vi "parse_dataString.vi"(4 "Timestamp":ext, 6 "Timebase Frequency":ext, 7 "Includes Timestamp?":bool=TRUE, 8 "error in (no error)":errorcluster, 9 "ChannelInfo":T2, 10 "Data Type":u32, 11 "Data String":string) -> (0 "error out":errorcluster, 3 "Data":T1)   [LabVIEW 2020, in "OXYGEN_Datastream.lvlib"]
uses:
  OXYGEN_Datastream.lvlib
  TypeDefs/ChannelInfo.ctl
  TypeDefs/ChannelInfo_Scaling.ctl
  TypeDefs/DataPoint_Variant.ctl
  TypeDefs/CAN_Data.ctl
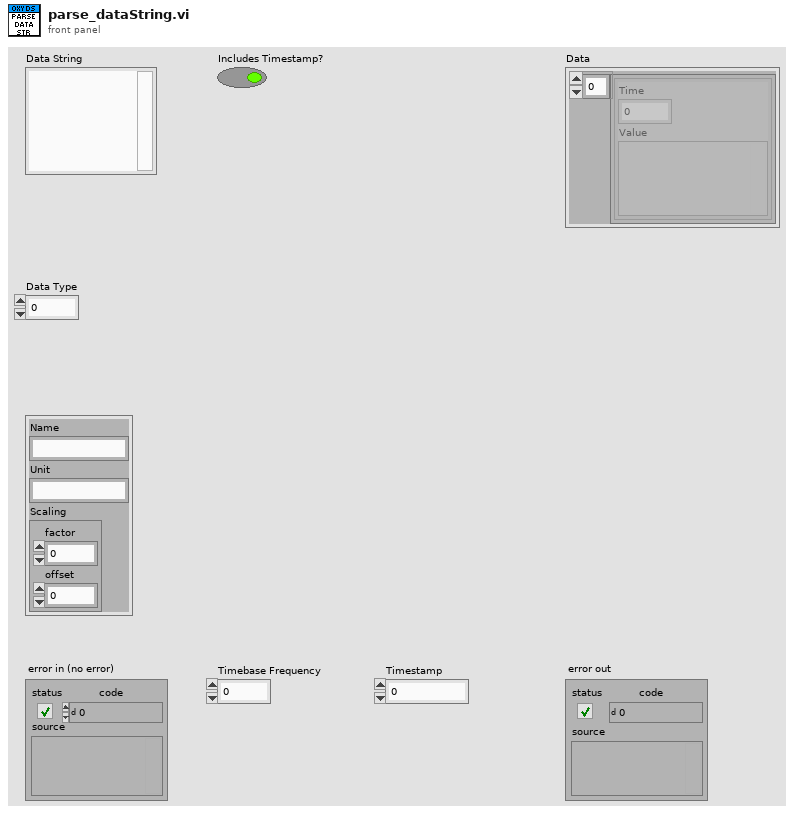
[diagram p1: front panel]
types:
  T1 = typedef "OXYGEN_Datastream.lvlib/DataPoint_Variant.ctl" = cluster{"DataPoints":cluster{"Time":dbl, "Value":variant}[]}
  T2 = typedef "OXYGEN_Datastream.lvlib/ChannelInfo.ctl" = cluster{"Name":string, "Unit":string, "Scaling":T3}
  T3 = typedef "OXYGEN_Datastream.lvlib/ChannelInfo_Scaling.ctl" = cluster{"factor":dbl, "offset":dbl}
  T4 = enum16{"big-endian, network order", "native, host order", "little-endian"}
  T5 = typedef "OXYGEN_Datastream.lvlib/CAN_Data.ctl" = cluster{"ID":string, "Message":string}
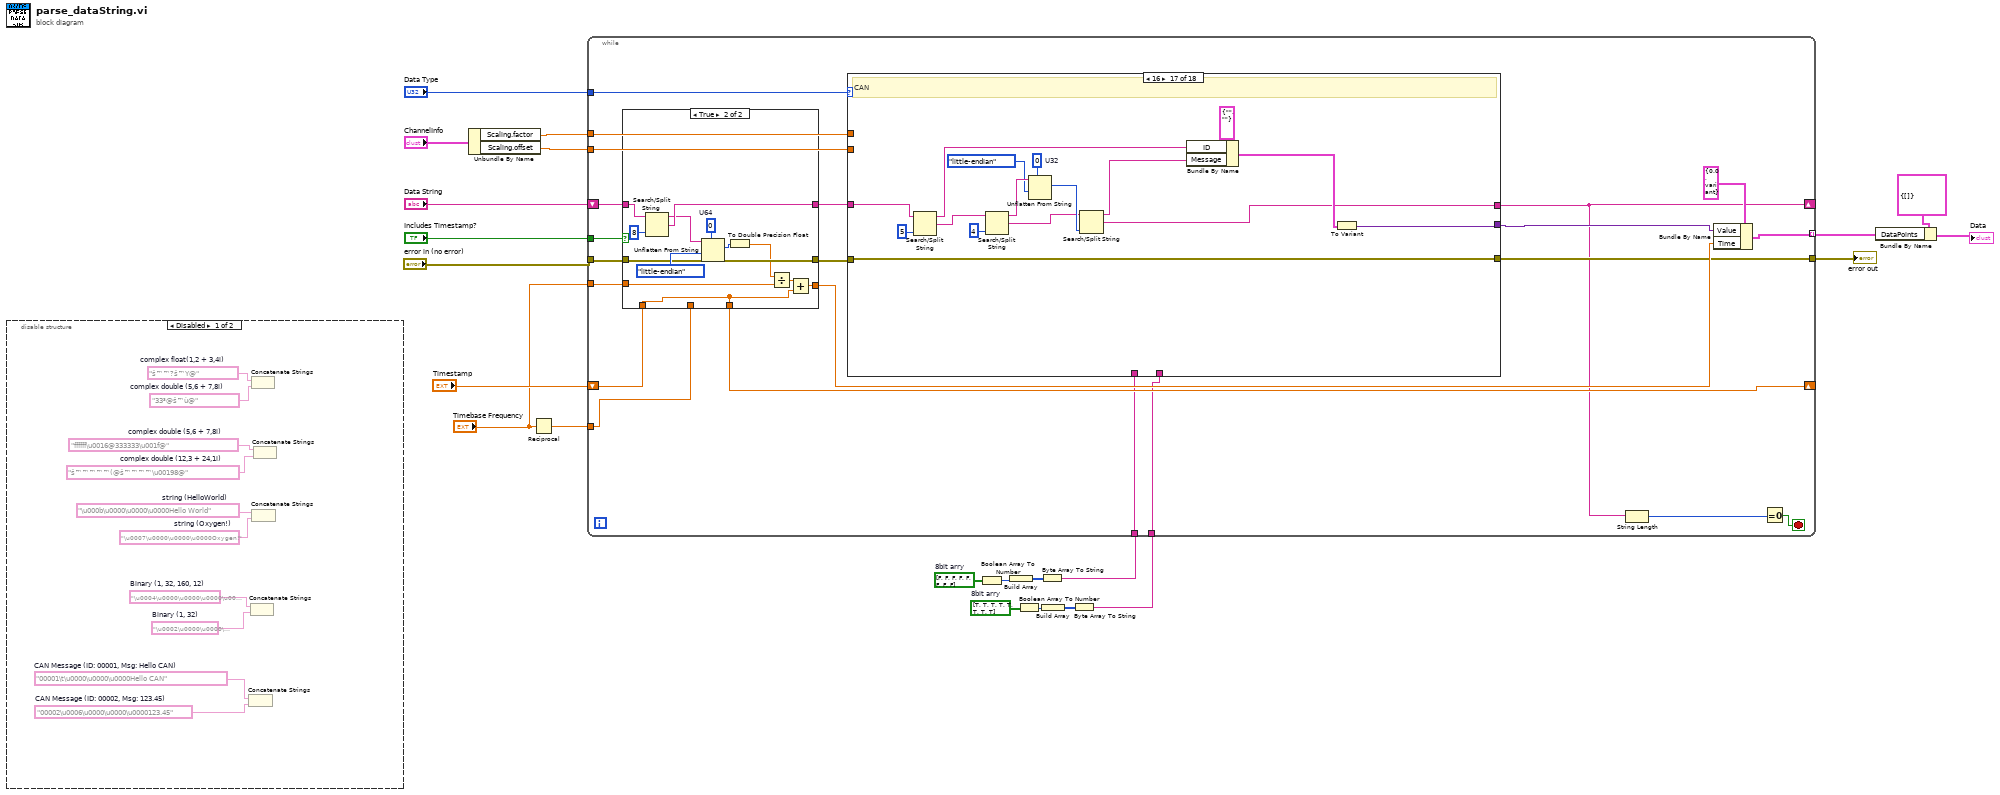
[diagram p0: block diagram]
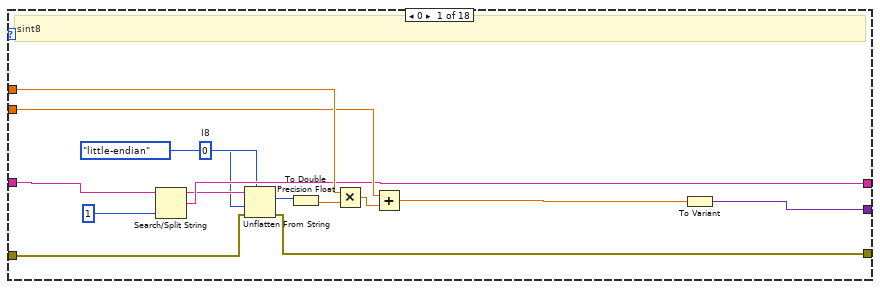
[diagram p3: hidden frame]
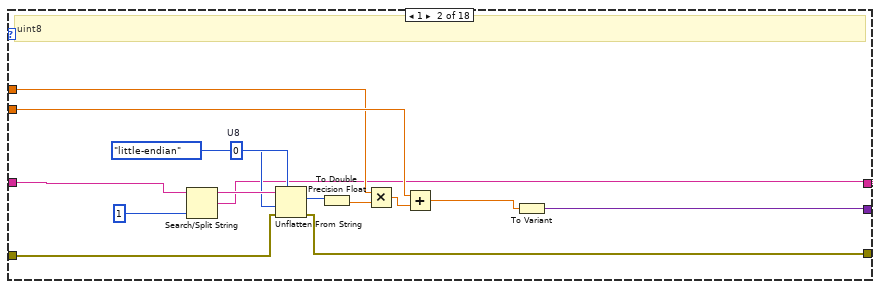
[diagram p4: hidden frame]
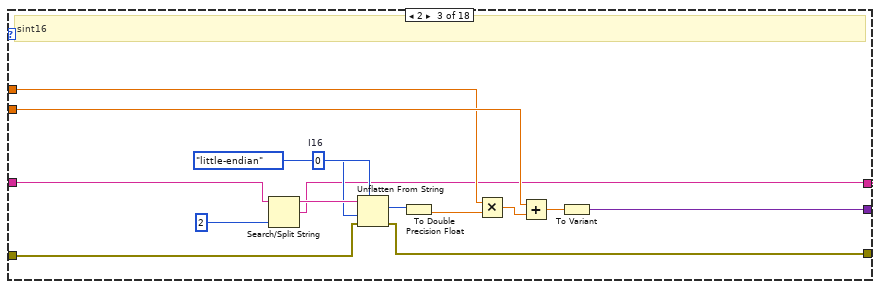
[diagram p5: hidden frame]
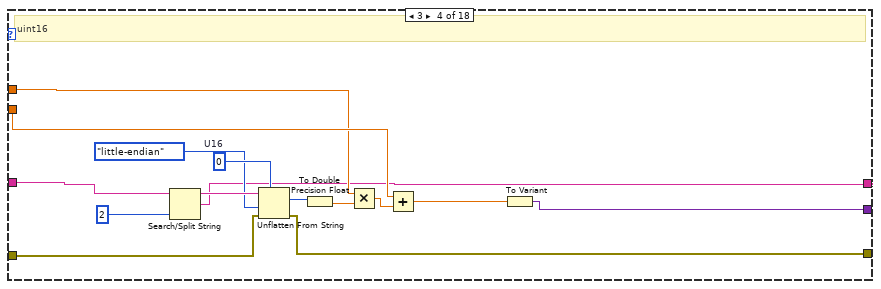
[diagram p6: hidden frame]
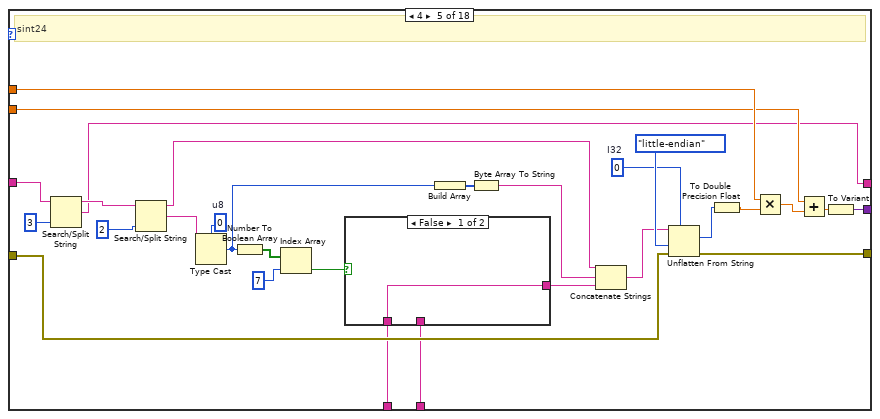
[diagram p7: hidden frame]
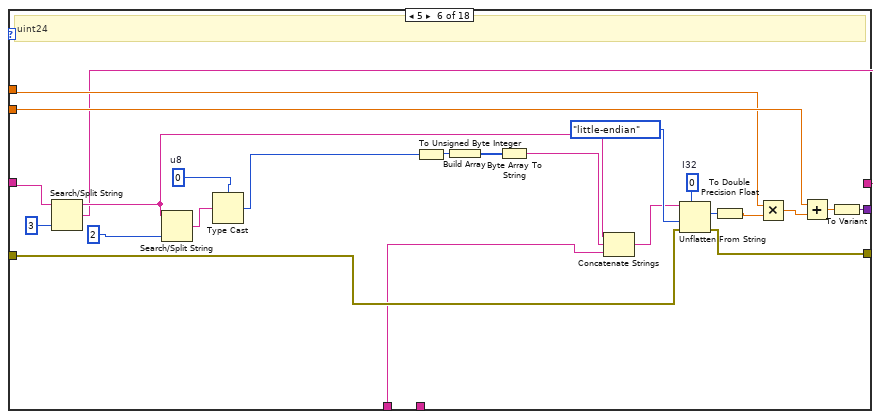
[diagram p9: hidden frame]
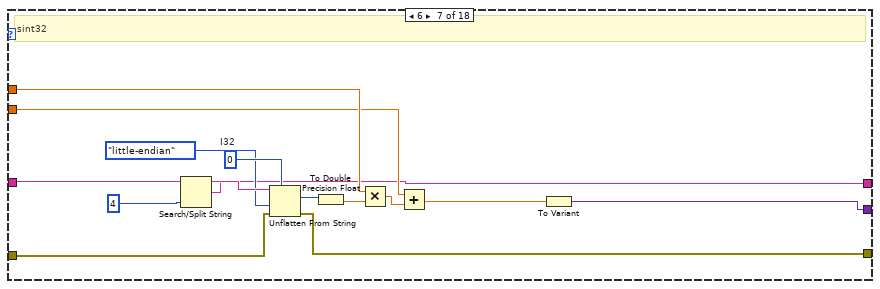
[diagram p10: hidden frame]
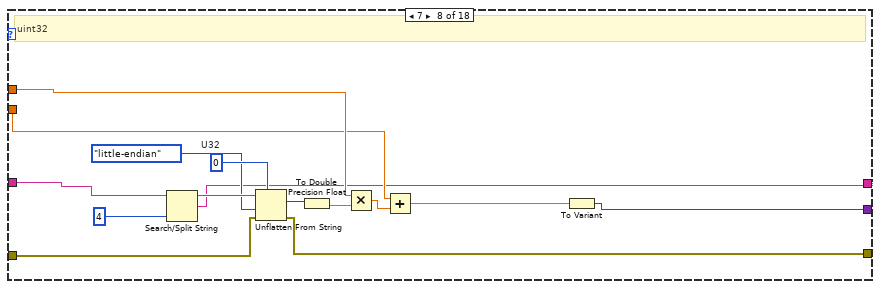
[diagram p11: hidden frame]
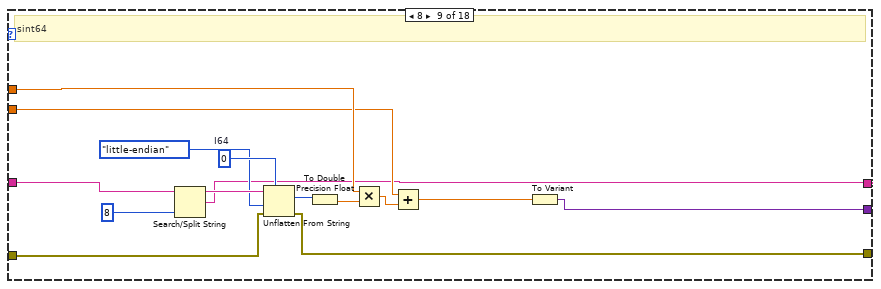
[diagram p12: hidden frame]
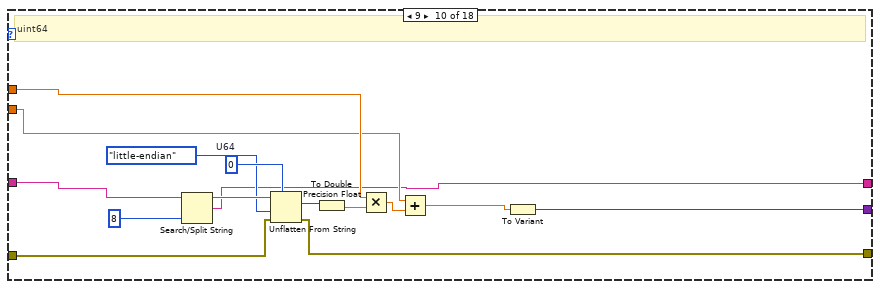
[diagram p13: hidden frame]
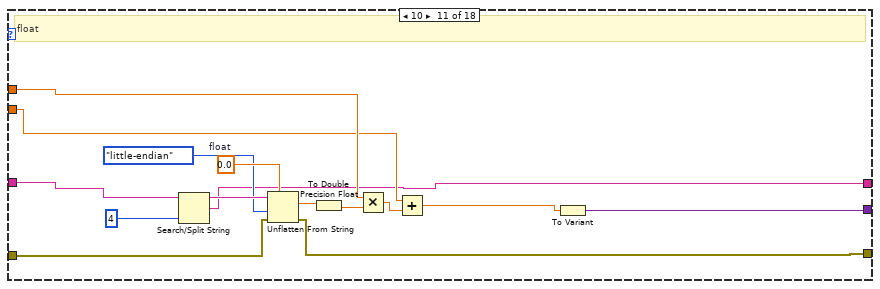
[diagram p14: hidden frame]
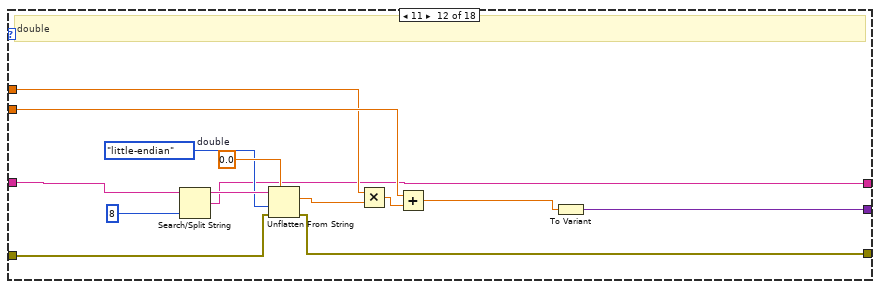
[diagram p15: hidden frame]
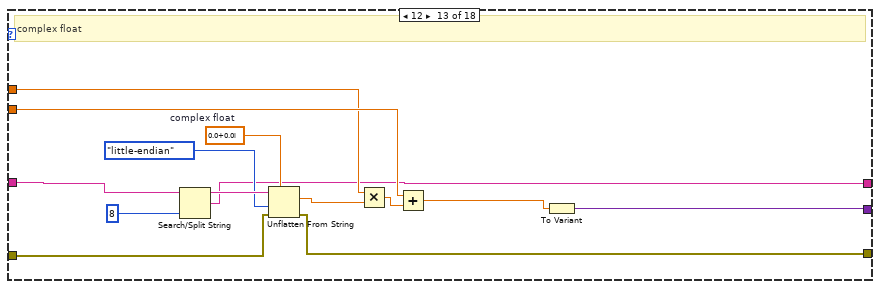
[diagram p16: hidden frame]
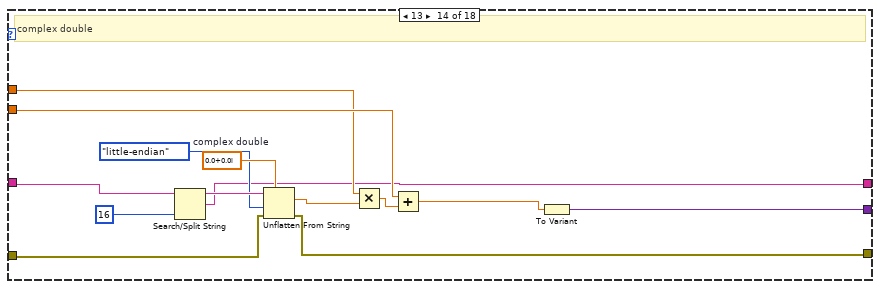
[diagram p17: hidden frame]
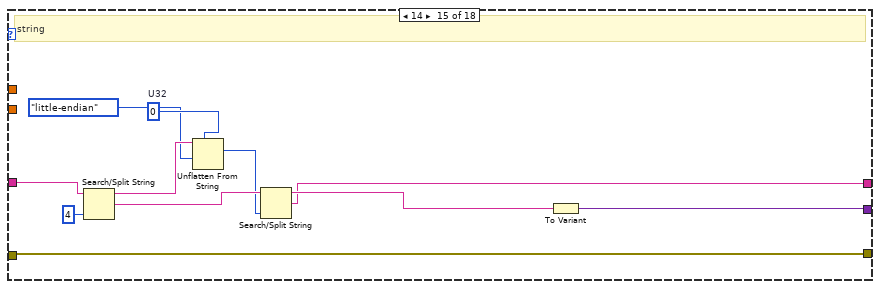
[diagram p18: hidden frame]
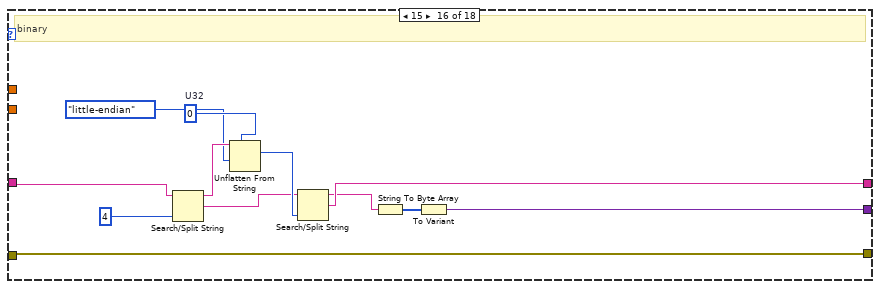
[diagram p19: hidden frame]
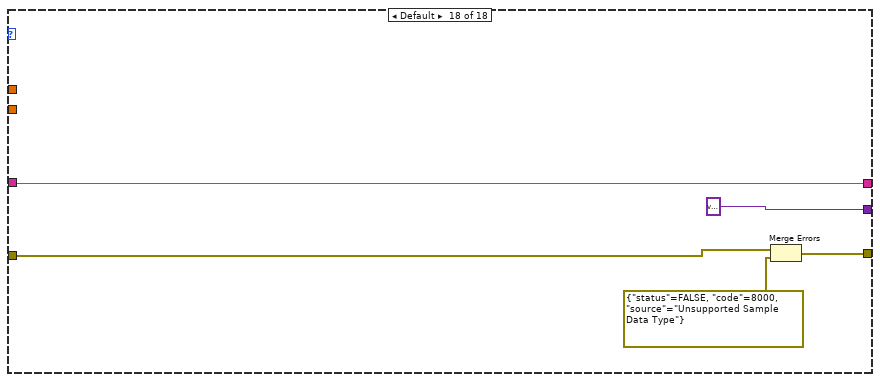
[diagram p20: hidden frame]
diagram:
  w8 = bool[] [TRUE, TRUE, TRUE, TRUE, TRUE, TRUE, TRUE, TRUE]  # 8bit arry
  w9 = bool[] [FALSE, FALSE, FALSE, FALSE, FALSE, FALSE, FALSE, FALSE]  # 8bit arry
  n1 = disable-structure shown="Disabled" {
    frame Disabled {
      w23 = "00002\u0006\u0000\u0000\u0000123.45"  # CAN Message (ID: 00002, Msg: 123.45)
      w24 = "00001\t\u0000\u0000\u0000Hello CAN"  # CAN Message (ID: 00001, Msg: Hello CAN)
      w25 = "\u0002\u0000\u0000\u0000\u0001 "  # Binary (1, 32)
      w26 = "\u0004\u0000\u0000\u0000\u0001  \f"  # Binary (1, 32, 160, 12)
      w27 = "š™™™™™(@š™™™™\u00198@"  # complex double (12,3 + 24,1i)
      w29 = "33³@š™ù@"  # complex double (5,6 + 7,8i)
      w31 = "\u0007\u0000\u0000\u0000Oxygen!"  # string (Oxygen!)
      w32 = "\u000b\u0000\u0000\u0000Hello World"  # string (HelloWorld)
      w28 = "ffffff\u0016@333333\u001f@"  # complex double (5,6 + 7,8i)
      w30 = "š™™?š™Y@"  # complex float(1,2 + 3,4i)
      n2 = Concatenate Strings(w24, w23) -> ()  [unwired: 1 out]
      n3 = Concatenate Strings(w26, w25) -> ()  [unwired: 1 out]
      n4 = Concatenate Strings(w30, w29) -> ()  [unwired: 1 out]
      n5 = Concatenate Strings(w32, w31) -> ()  [unwired: 1 out]
      n6 = Concatenate Strings(w28, w27) -> ()  [unwired: 1 out]
    }
    frame Enabled {
    }
  }
  n7 = Unbundle By Name("ChannelInfo") -> ("Scaling.factor"=w19:dbl, "Scaling.offset"=w18:dbl)
  n8 = Reciprocal(x="Timebase Frequency") -> (1/x=w10:ext)
  n9 = Boolean Array To Number(Boolean array=w9) -> (number=w7:u32)
  n10 = Build Array(w7) -> (w6:u32[])
  n11 = Boolean Array To Number(Boolean array=w8) -> (number=w5:u32)
  n12 = Byte Array To String(unsigned byte array=w6) -> (string=w3:string)
  n13 = Build Array(w5) -> (w4:u32[])
  n14 = Byte Array To String(unsigned byte array=w4) -> (string=w2:string)
  n15 = while {
    tunnel: "Data Type" -> [w39]
    tunnel: w19 -> [w40]
    tunnel: w18 -> [w41]
    shift-right: [w36] -> _
    shift-left: "Data String" -> [w52]
    tunnel: "Includes Timestamp?" -> [w48]
    tunnel: "error in (no error)" -> [w51]
    tunnel: [w38] -> w16
    tunnel: [w49] -> w12 mode=indexing
    shift-right: [w44] -> _
    shift-left: "Timestamp" -> [w47]
    tunnel: w10 -> [w46]
    tunnel: w3 -> [w35]
    tunnel: w2 -> [w34]
    tunnel: "Timebase Frequency" -> [w33]
    stop <- w53 stop-if-true
    n16 = case shown="True" w48 {
      tunnel: w52 -> [w335 w348]
      tunnel: [w335 w347] -> w42
      tunnel: [w332 w338] -> w45
      tunnel: [w334 w342] -> w43
      tunnel: w51 -> [w334 w341]
      tunnel: w47 -> [w332 w337]
      tunnel: w46 -> [w333 _]
      tunnel: [w331 w337] -> w44
      tunnel: w33 -> [_ w336]
      frame False {
        n17 = Add(x=w332, y=w333) -> (x+y=w331:ext)
      }
      frame True {
        w345 = u64 0  # U64
        n18 = Search/Split String(string=w348, offset (0)=8) -> (substring before match=w346:string, match + rest of string=w347:string)  [unwired: 1 in, 1 out]
        n19 = Unflatten From String(type=w345, binary string=w346, byte order (0:big-endian, network order)=T4."little-endian", error in (no error)=w341) -> (value=w343:u64, error out=w342:errorcluster)  [unwired: 1 in, 1 out]
        n20 = To Double Precision Float(number=w343) -> (double precision float=w339:dbl)
        n21 = Divide(x=w339, y=w336) -> (x/y=w340:ext)
        n22 = Add(x=w340, y=w337) -> (x+y=w338:ext)
      }
    }
    n23 = case shown="16" w39 {
      tunnel: w42 -> [w69 w84 w99 w114 w143 w169 w182 w197 w212 w227 w242 w258 w272 w278 w294 w302 w317 w330]
      tunnel: [w55 w70 w85 w100 w121 w151 w171 w185 w200 w215 w230 w245 w259 w274 w297 w298 w313 variant] -> w37
      tunnel: w40 -> [w68 w82 w97 w112 w142 w167 w184 w199 w214 w229 w244 w256 w270 w276 _ _ _ _]
      tunnel: w41 -> [w67 w83 w98 w113 w141 w168 w183 w198 w213 w228 w243 w257 w271 w277 _ _ _ _]
      tunnel: [w66 w74 w89 w104 w125 w155 w174 w189 w204 w219 w234 w249 w263 w275 w287 w301 w311 w330] -> w36
      tunnel: w43 -> [w58 w73 w88 w103 w124 w154 w173 w187 w202 w217 w232 w247 w261 w279 w296 w309 w325 w328]
      tunnel: [w57 w72 w87 w102 w123 w153 w172 w188 w203 w218 w233 w248 w262 w273 w296 w309 w325 w329] -> w38
      tunnel: w35 -> [_ _ _ _ w120 w150 _ _ _ _ _ _ _ _ _ _ _ _]
      tunnel: w34 -> [_ _ _ _ w119 _ _ _ _ _ _ _ _ _ _ _ _ _]
      frame 0 {
        w63 = i8 0  # I8
        # "sint8"
        n24 = Search/Split String(string=w69, offset (0)=1) -> (substring before match=w64:string, match + rest of string=w66:string)  [unwired: 1 in, 1 out]
        n25 = Unflatten From String(type=w63, binary string=w64, byte order (0:big-endian, network order)=T4."little-endian", error in (no error)=w58) -> (value=w61:i8, error out=w57:errorcluster)  [unwired: 1 in, 1 out]
        n26 = To Double Precision Float(number=w61) -> (double precision float=w60:dbl)
        n27 = Multiply(x=w68, y=w60) -> (x*y=w59:dbl)
        n28 = Add(x=w67, y=w59) -> (x+y=w56:dbl)
        n29 = To Variant(anything=w56) -> (Variant=w55:variant)
      }
      frame 1 {
        w79 = u8 0  # U8
        # "uint8"
        n30 = Search/Split String(string=w84, offset (0)=1) -> (substring before match=w80:string, match + rest of string=w74:string)  [unwired: 1 in, 1 out]
        n31 = Unflatten From String(type=w79, binary string=w80, byte order (0:big-endian, network order)=T4."little-endian", error in (no error)=w73) -> (value=w77:u8, error out=w72:errorcluster)  [unwired: 1 in, 1 out]
        n32 = To Double Precision Float(number=w77) -> (double precision float=w76:dbl)
        n33 = Multiply(x=w82, y=w76) -> (x*y=w75:dbl)
        n34 = Add(x=w83, y=w75) -> (x+y=w71:dbl)
        n35 = To Variant(anything=w71) -> (Variant=w70:variant)
      }
      frame 2 {
        w94 = i16 0  # I16
        # "sint16"
        n36 = Search/Split String(string=w99, offset (0)=2) -> (substring before match=w95:string, match + rest of string=w89:string)  [unwired: 1 in, 1 out]
        n37 = Unflatten From String(type=w94, binary string=w95, byte order (0:big-endian, network order)=T4."little-endian", error in (no error)=w88) -> (value=w92:i16, error out=w87:errorcluster)  [unwired: 1 in, 1 out]
        n38 = To Double Precision Float(number=w92) -> (double precision float=w91:dbl)
        n39 = Multiply(x=w97, y=w91) -> (x*y=w90:dbl)
        n40 = Add(x=w98, y=w90) -> (x+y=w86:dbl)
        n41 = To Variant(anything=w86) -> (Variant=w85:variant)
      }
      frame 3 {
        w109 = u16 0  # U16
        # "uint16"
        n42 = Search/Split String(string=w114, offset (0)=2) -> (substring before match=w110:string, match + rest of string=w104:string)  [unwired: 1 in, 1 out]
        n43 = Unflatten From String(type=w109, binary string=w110, byte order (0:big-endian, network order)=T4."little-endian", error in (no error)=w103) -> (value=w107:u16, error out=w102:errorcluster)  [unwired: 1 in, 1 out]
        n44 = To Double Precision Float(number=w107) -> (double precision float=w106:dbl)
        n45 = Multiply(x=w112, y=w106) -> (x*y=w105:dbl)
        n46 = Add(x=w113, y=w105) -> (x+y=w101:dbl)
        n47 = To Variant(anything=w101) -> (Variant=w100:variant)
      }
      frame 4 {
        w131 = u8 0  # u8
        w135 = 0  # I32
        # "sint24"
        n48 = Search/Split String(string=w143, offset (0)=3) -> (substring before match=w133:string, match + rest of string=w125:string)  [unwired: 1 in, 1 out]
        n49 = Search/Split String(string=w133, offset (0)=2) -> (substring before match=w129:string, match + rest of string=w132:string)  [unwired: 1 in, 1 out]
        n50 = Type Cast(type=w131, x=w132) -> (*(type *) &x=w115:u8)
        n51 = Number To Boolean Array(number=w115) -> (Boolean array=w126:bool[])
        n52 = Index Array(array=w126, index=7) -> (element=w127:bool)
        n53 = case shown="False" w127 {
          tunnel: [w144 w145] -> w118
          tunnel: w120 -> [w144 _]
          tunnel: w119 -> [_ w145]
          frame False {
          }
          frame True {
          }
        }
        n54 = Build Array(w115) -> (w117:u8[])
        n55 = Byte Array To String(unsigned byte array=w117) -> (string=w116:string)
        n56 = Concatenate Strings(w129, w116, w118) -> (w128:string)
        n57 = Unflatten From String(type=w135, binary string=w128, byte order (0:big-endian, network order)=T4."little-endian", error in (no error)=w124) -> (value=w136:i32, error out=w123:errorcluster)  [unwired: 1 in, 1 out]
        n58 = To Double Precision Float(number=w136) -> (double precision float=w138:dbl)
        n59 = Multiply(x=w142, y=w138) -> (x*y=w137:dbl)
        n60 = Add(x=w141, y=w137) -> (x+y=w122:dbl)
        n61 = To Variant(anything=w122) -> (Variant=w121:variant)
      }
      frame 5 {
        w158 = u8 0  # u8
        w161 = u32 0  # I32
        # "uint24"
        n62 = Search/Split String(string=w169, offset (0)=3) -> (substring before match=w156:string, match + rest of string=w155:string)  [unwired: 1 in, 1 out]
        n63 = Search/Split String(string=w156, offset (0)=2) -> (match + rest of string=w159:string)  [unwired: 1 in, 2 out]
        n64 = Type Cast(type=w158, x=w159) -> (*(type *) &x=w146:u8)
        n65 = To Unsigned Byte Integer(number=w146) -> (unsigned 8bit integer=w147:u8)
        n66 = Build Array(w147) -> (w149:u8[])
        n67 = Byte Array To String(unsigned byte array=w149) -> (string=w148:string)
        n68 = Concatenate Strings(w156, w148, w150) -> (w157:string)
        n69 = Unflatten From String(type=w161, binary string=w157, byte order (0:big-endian, network order)=T4."little-endian", error in (no error)=w154) -> (value=w162:u32, error out=w153:errorcluster)  [unwired: 1 in, 1 out]
        n70 = To Double Precision Float(number=w162) -> (double precision float=w164:dbl)
        n71 = Multiply(x=w167, y=w164) -> (x*y=w163:dbl)
        n72 = Add(x=w168, y=w163) -> (x+y=w152:dbl)
        n73 = To Variant(anything=w152) -> (Variant=w151:variant)
      }
      frame 6 {
        w179 = 0  # I32
        # "sint32"
        n74 = Search/Split String(string=w182, offset (0)=4) -> (substring before match=w180:string, match + rest of string=w174:string)  [unwired: 1 in, 1 out]
        n75 = Unflatten From String(type=w179, binary string=w180, byte order (0:big-endian, network order)=T4."little-endian", error in (no error)=w173) -> (value=w177:i32, error out=w172:errorcluster)  [unwired: 1 in, 1 out]
        n76 = To Double Precision Float(number=w177) -> (double precision float=w176:dbl)
        n77 = Multiply(x=w184, y=w176) -> (x*y=w175:dbl)
        n78 = Add(x=w183, y=w175) -> (x+y=w170:dbl)
        n79 = To Variant(anything=w170) -> (Variant=w171:variant)
      }
      frame 7 {
        w194 = u32 0  # U32
        # "uint32"
        n80 = Search/Split String(string=w197, offset (0)=4) -> (substring before match=w195:string, match + rest of string=w189:string)  [unwired: 1 in, 1 out]
        n81 = Unflatten From String(type=w194, binary string=w195, byte order (0:big-endian, network order)=T4."little-endian", error in (no error)=w187) -> (value=w192:u32, error out=w188:errorcluster)  [unwired: 1 in, 1 out]
        n82 = To Double Precision Float(number=w192) -> (double precision float=w191:dbl)
        n83 = Multiply(x=w199, y=w191) -> (x*y=w190:dbl)
        n84 = Add(x=w198, y=w190) -> (x+y=w186:dbl)
        n85 = To Variant(anything=w186) -> (Variant=w185:variant)
      }
      frame 8 {
        w209 = i64 0  # I64
        # "sint64"
        n86 = Search/Split String(string=w212, offset (0)=8) -> (substring before match=w210:string, match + rest of string=w204:string)  [unwired: 1 in, 1 out]
        n87 = Unflatten From String(type=w209, binary string=w210, byte order (0:big-endian, network order)=T4."little-endian", error in (no error)=w202) -> (value=w207:i64, error out=w203:errorcluster)  [unwired: 1 in, 1 out]
        n88 = To Double Precision Float(number=w207) -> (double precision float=w206:dbl)
        n89 = Multiply(x=w214, y=w206) -> (x*y=w205:dbl)
        n90 = Add(x=w213, y=w205) -> (x+y=w201:dbl)
        n91 = To Variant(anything=w201) -> (Variant=w200:variant)
      }
      frame 9 {
        w224 = u64 0  # U64
        # "uint64"
        n92 = Search/Split String(string=w227, offset (0)=8) -> (substring before match=w225:string, match + rest of string=w219:string)  [unwired: 1 in, 1 out]
        n93 = Unflatten From String(type=w224, binary string=w225, byte order (0:big-endian, network order)=T4."little-endian", error in (no error)=w217) -> (value=w222:u64, error out=w218:errorcluster)  [unwired: 1 in, 1 out]
        n94 = To Double Precision Float(number=w222) -> (double precision float=w221:dbl)
        n95 = Multiply(x=w229, y=w221) -> (x*y=w220:dbl)
        n96 = Add(x=w228, y=w220) -> (x+y=w216:dbl)
        n97 = To Variant(anything=w216) -> (Variant=w215:variant)
      }
      frame 10 {
        w239 = sgl 0.0  # float
        # "float"
        n98 = Search/Split String(string=w242, offset (0)=4) -> (substring before match=w240:string, match + rest of string=w234:string)  [unwired: 1 in, 1 out]
        n99 = Unflatten From String(type=w239, binary string=w240, byte order (0:big-endian, network order)=T4."little-endian", error in (no error)=w232) -> (value=w237:sgl, error out=w233:errorcluster)  [unwired: 1 in, 1 out]
        n100 = To Double Precision Float(number=w237) -> (double precision float=w236:dbl)
        n101 = Multiply(x=w244, y=w236) -> (x*y=w235:dbl)
        n102 = Add(x=w243, y=w235) -> (x+y=w231:dbl)
        n103 = To Variant(anything=w231) -> (Variant=w230:variant)
      }
      frame 11 {
        w253 = 0.0  # double
        # "double"
        n104 = Search/Split String(string=w258, offset (0)=8) -> (substring before match=w254:string, match + rest of string=w249:string)  [unwired: 1 in, 1 out]
        n105 = Unflatten From String(type=w253, binary string=w254, byte order (0:big-endian, network order)=T4."little-endian", error in (no error)=w247) -> (value=w250:dbl, error out=w248:errorcluster)  [unwired: 1 in, 1 out]
        n106 = Multiply(x=w256, y=w250) -> (x*y=w251:dbl)
        n107 = Add(x=w257, y=w251) -> (x+y=w246:dbl)
        n108 = To Variant(anything=w246) -> (Variant=w245:variant)
      }
      frame 12 {
        w267 = csg 0.0+0.0i  # complex float
        # "complex float"
        n109 = Search/Split String(string=w272, offset (0)=8) -> (substring before match=w268:string, match + rest of string=w263:string)  [unwired: 1 in, 1 out]
        n110 = Unflatten From String(type=w267, binary string=w268, byte order (0:big-endian, network order)=T4."little-endian", error in (no error)=w261) -> (value=w264:csg, error out=w262:errorcluster)  [unwired: 1 in, 1 out]
        n111 = Multiply(x=w270, y=w264) -> (x*y=w265:cdb)
        n112 = Add(x=w271, y=w265) -> (x+y=w260:cdb)
        n113 = To Variant(anything=w260) -> (Variant=w259:variant)
      }
      frame 13 {
        w284 = cdb 0.0+0.0i  # complex double
        # "complex double"
        n114 = Search/Split String(string=w278, offset (0)=16) -> (substring before match=w285:string, match + rest of string=w275:string)  [unwired: 1 in, 1 out]
        n115 = Unflatten From String(type=w284, binary string=w285, byte order (0:big-endian, network order)=T4."little-endian", error in (no error)=w279) -> (value=w281:cdb, error out=w273:errorcluster)  [unwired: 1 in, 1 out]
        n116 = Multiply(x=w276, y=w281) -> (x*y=w282:cdb)
        n117 = Add(x=w277, y=w282) -> (x+y=w280:cdb)
        n118 = To Variant(anything=w280) -> (Variant=w274:variant)
      }
      frame 14 {
        w291 = u32 0  # U32
        # "string"
        n119 = Search/Split String(string=w294, offset (0)=4) -> (substring before match=w292:string, match + rest of string=w293:string)  [unwired: 1 in, 1 out]
        n120 = Unflatten From String(type=w291, binary string=w292, byte order (0:big-endian, network order)=T4."little-endian") -> (value=w289:u32)  [unwired: 2 in, 2 out]
        n121 = Search/Split String(string=w293, offset (0)=w289) -> (substring before match=w288:string, match + rest of string=w287:string)  [unwired: 1 in, 1 out]
        n122 = To Variant(anything=w288) -> (Variant=w297:variant)
      }
      frame 15 {
        w305 = u32 0  # U32
        # "binary"
        n123 = Search/Split String(string=w302, offset (0)=4) -> (substring before match=w307:string, match + rest of string=w306:string)  [unwired: 1 in, 1 out]
        n124 = Unflatten From String(type=w305, binary string=w307, byte order (0:big-endian, network order)=T4."little-endian") -> (value=w308:u32)  [unwired: 2 in, 2 out]
        n125 = Search/Split String(string=w306, offset (0)=w308) -> (substring before match=w300:string, match + rest of string=w301:string)  [unwired: 1 in, 1 out]
        n126 = String To Byte Array(string=w300) -> (unsigned byte array=w299:u8[])
        n127 = To Variant(anything=w299) -> (Variant=w298:variant)
      }
      frame 16 {
        w321 = u32 0  # U32
        # "CAN"
        n128 = Search/Split String(string=w317, offset (0)=5) -> (substring before match=w315:string, match + rest of string=w316:string)  [unwired: 1 in, 1 out]
        n129 = Search/Split String(string=w316, offset (0)=4) -> (substring before match=w323:string, match + rest of string=w322:string)  [unwired: 1 in, 1 out]
        n130 = Unflatten From String(type=w321, binary string=w323, byte order (0:big-endian, network order)=T4."little-endian") -> (value=w324:u32)  [unwired: 2 in, 2 out]
        n131 = Search/Split String(string=w322, offset (0)=w324) -> (substring before match=w312:string, match + rest of string=w311:string)  [unwired: 1 in, 1 out]
        n132 = Bundle By Name(cluster=T5 {"ID"="", "Message"=""} ("CAN_Data"), "ID"=w315, "Message"=w312) -> (w314:T5)
        n133 = To Variant(anything=w314) -> (Variant=w313:variant)
      }
      frame Default {
        n134 = Merge Errors(w328, errorcluster {"status"=FALSE, "code"=8000, "source"="Unsupported Sample Data Type"} ("error in")) -> (w329:errorcluster)
      }
    }
    n135 = String Length(string=w36) -> (length=w54:i32)
    n136 = Bundle By Name(cluster=cluster{"Time":dbl, "Value":variant} {"Time"=0.0, "Value"=variant}, "Value"=w37, "Time"=w45) -> (w49:cluster{"Time":dbl, "Value":variant})
    n137 = Equal To 0?(x=w54) -> (x = 0?=w53:bool)
  }
  "error out" <- w16
  n138 = Bundle By Name(cluster=T1 {"DataPoints"=[]} ("Data"), "DataPoints"=w12) -> (→"Data":T1)
